vi "Status USB Address.vi"(5 "Retry Attempts (0)":i32 min=0, 7 "Unit Address (-1)":i32=-1, 8 "error in (no error)":errorcluster, 11 "VISA resource name (in)":refnum<visa-resource-name>) -> (0 "error out":errorcluster, 2 "Address":i32, 3 "VISA resource name (out)":refnum<visa-resource-name>)   [LabVIEW 2020, in "Omega Platinum Series.lvlib"]
doc: "Gets the address for the controller though USB connection."
uses:
  Omega Platinum Series.lvlib
panel:
  out "Command":string
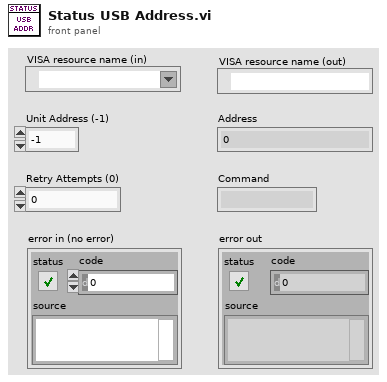
[diagram p1: front panel]
types:
  T1 = typedef "Omega Platinum Series.lvlib/Response.ctl" = cluster{"Unit Address":i32, "Command Class":string, "Command ID":u32, "Parameters":string}
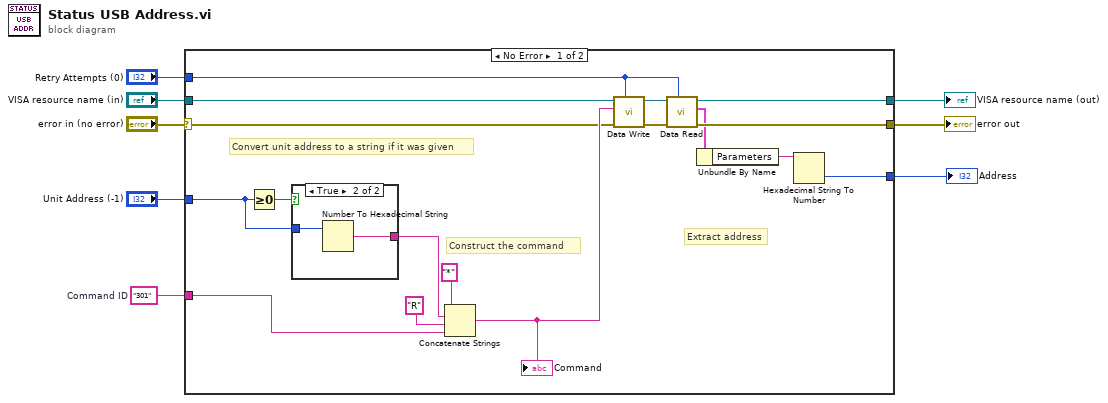
[diagram p0: block diagram]
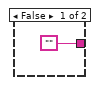
[diagram p2: hidden frame]
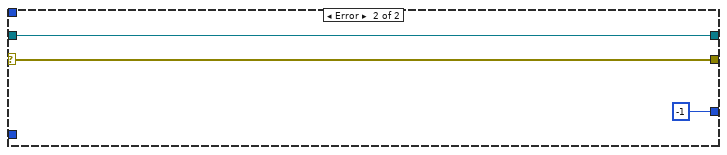
[diagram p3: hidden frame]
diagram:
  w8 = "301"  # Command ID
  n1 = case shown="No Error" "error in (no error)" {
    selector: "error in (no error)" -> [w19 w31]
    tunnel: w8 -> [w13 _]
    tunnel: "Unit Address (-1)" -> [w23 _]
    tunnel: [w15 w31] -> w5
    tunnel: "VISA resource name (in)" -> [w21 w30]
    tunnel: [w16 w30] -> w3
    tunnel: [w10 -1] -> w2
    tunnel: "Retry Attempts (0)" -> [w9 _]
    frame No Error {
      # "Extract address"
      # "Convert unit address to a string if it was given"
      # "Construct the command"
      n2 = Greater Or Equal To 0?(x=w23) -> (x >= 0?=w25:bool)
      n3 = case shown="True" w25 {
        tunnel: w23 -> [_ w28]
        tunnel: ["" w27] -> w22
        frame False {
        }
        frame True {
          n4 = Number To Hexadecimal String(2:w28) -> (0:w27:string)  [unwired: 1 in]
        }
      }
      n5 = Concatenate Strings("*" ("string"), w22, "R" ("string"), w13) -> (w20:string)
      "Command" <- w20
      n6 = call "Data Write.vi"("Retry Attempts (0)"=w9, "error in (no error)"=w19, "Command"=w20, "VISA Refnum in"=w21) -> ("error out"=w18:errorcluster, "VISA Refnum out"=w17:refnum<visa-resource-name>)  [unwired: 6 in]
      n7 = call "Data Read.vi"("Retry Attempts (0)"=w9, "error in (no error)"=w18, "VISA Refnum in"=w17) -> ("error out"=w15:errorcluster, "Response Cluster"=w12:T1, "VISA Refnum out"=w16:refnum<visa-resource-name>)  [unwired: 5 in, 1 out]
      n8 = Unbundle By Name(w12) -> ("Parameters"=w11:string)
      n9 = Hexadecimal String To Number(string=w11) -> (number=w10:u32)  [unwired: 2 in, 1 out]
    }
    frame Error {
    }
  }
  "error out" <- w5
  "VISA resource name (out)" <- w3
  "Address" <- w2
